vi "Autonomous Independent.vi"() -> ()   [LabVIEW 2017]
doc: "This VI is called when autonomous begins, and will automatically be terminated when autonomous ends. You can carry out timed or sensor driven robot movement independently without needing to return to the caller."
uses:
  Auto Movement Cluster.ctl
  Begin Cluster.ctl
  <vilib>/Rock Robotics/WPI/Encoder/WPI_EncoderDevRef.ctl
  <vilib>/Rock Robotics/SystemInterfaces/Encoder/FPGA_EncoderIdx.ctl
  <vilib>/Rock Robotics/SystemInterfaces/Counter/FPGA_CounterCtrSystemIndex.ctl
  <vilib>/Rock Robotics/WPI/Encoder/WPI_EncoderType.ctl
  <vilib>/Rock Robotics/WPI/Solenoid/WPI_SolenoidDevRef.ctl
  <vilib>/Rock Robotics/WPI/Solenoid/WPI_SolenoidChannel.ctl
  <vilib>/Rock Robotics/WPI/Potentiometer/WPI_PotentiometerDevRef.ctl
  <vilib>/Rock Robotics/SystemInterfaces/AI/FPGA_AIChannel.ctl
  <vilib>/Rock Robotics/WPI/Gyro/WPI_GyroDevRef.ctl
  <vilib>/Rock Robotics/SystemInterfaces/spilib/spi_bus.ctl
  <vilib>/Rock Robotics/WPI/RobotDrive/WPI_RobotDriveDevRef.ctl
  <vilib>/Rock Robotics/WPI/MotorControl/WPI_MotorControlDeviceRef.ctl
  <vilib>/Rock Robotics/WPI/MotorControl/WPI_MotorControlType.ctl
  <vilib>/Rock Robotics/SystemInterfaces/DIO/FPGA_DIOPWMChannel.ctl
  <vilib>/Rock Robotics/WPI/PWM/WPI_PWMDeadband.ctl
  <vilib>/Rock Robotics/SystemInterfaces/DIO/FPGA_DIOChannel.ctl
  <vilib>/Rock Robotics/WPI/Joystick/WPI_JoystickDevRef.ctl
  <vilib>/Rock Robotics/WPI/Joystick/WPI_JoystickDeviceEnum.ctl
  <vilib>/Rock Robotics/WPI/Utilities/WPI_GetSetVariantRefNum.vi
  <vilib>/Rock Robotics/Network Tables/NT Read Number.vi
  Global Variables.vi
  <vilib>/Rock Robotics/Network Tables/NT Read Boolean.vi
  <vilib>/Rock Robotics/WPI/RobotDrive/WPI_RobotDriveArcadeDrive_Standard(NoSaturation).vi
panel:
  in  "SO - Switch & Scale":T1[](array[typedef])=[{"Drive "=-190.0, "Turn"=0.0, "Wait in ms"=0.0, "Turn?"=FALSE, "Wait?"=FALSE, "Align?"=FALSE, "Wait/Turn Drive Power"=0.0, "Wait Turn Power"=0.0, "Elevator Setpoint"=40.0, "Linear Actuator Length"=0.62, "Intake State 2"=enum."Off"}, {"Drive "=0.0, "Turn"=-90.0, "Wait in ms"=0.0, "Turn?"=TRUE, "Wait?"=FALSE, "Align?"=FALSE, "Wait/Turn Drive Power"=0.0, "Wait Turn Power"=0.0, "Elevator Setpoint"=40.0, "Linear Actuator Length"=0.33, "Intake State 2"=enum."Off"}, {"Drive "=60.0, "Turn"=-90.0, "Wait in ms"=0.0, "Turn?"=FALSE, "Wait?"=FALSE, "Align?"=FALSE, "Wait/Turn Drive Power"=0.0, "Wait Turn Power"=0.0, "Elevator Setpoint"=40.0, "Linear Actuator Length"=0.33, "Intake State 2"=enum."Off"}, {"Drive "=0.0, "Turn"=0.0, "Wait in ms"=0.0, "Turn?"=TRUE, "Wait?"=FALSE, "Align?"=FALSE, "Wait/Turn Drive Power"=0.0, "Wait Turn Power"=0.0, "Elevator Setpoint"=40.0, "Linear Actuator Length"=0.33, "Intake State 2"=enum."Off"}, {"Drive "=0.0, "Turn"=0.0, "Wait in ms"=750.0, "Turn?"=FALSE, "Wait?"=TRUE, "Align?"=FALSE, "Wait/Turn Drive Power"=-0.5, "Wait Turn Power"=0.0, "Elevator Setpoint"=40.0, "Linear Actuator Length"=0.33, "Intake State 2"=enum."Off"}, {"Drive "=0.0, "Turn"=0.0, "Wait in ms"=500.0, "Turn?"=FALSE, "Wait?"=TRUE, "Align?"=FALSE, "Wait/Turn Drive Power"=0.0, "Wait Turn Power"=0.0, "Elevator Setpoint"=40.0, "Linear Actuator Length"=0.33, "Intake State 2"=enum."Spit High"}, {"Drive "=-50.0, "Turn"=-0.0, "Wait in ms"=0.0, "Turn?"=FALSE, "Wait?"=FALSE, "Align?"=FALSE, "Wait/Turn Drive Power"=0.0, "Wait Turn Power"=0.0, "Elevator Setpoint"=30.0, "Linear Actuator Length"=0.62, "Intake State 2"=enum."Off"}, {"Drive "=0.0, "Turn"=0.0, "Wait in ms"=1500.0, "Turn?"=FALSE, "Wait?"=FALSE, "Align?"=TRUE, "Wait/Turn Drive Power"=-0.5, "Wait Turn Power"=0.0, "Elevator Setpoint"=1.0, "Linear Actuator Length"=0.62, "Intake State 2"=enum."Intake"}, {"Drive "=-40.0, "Turn"=-0.0, "Wait in ms"=0.0, "Turn?"=FALSE, "Wait?"=FALSE, "Align?"=FALSE, "Wait/Turn Drive Power"=0.0, "Wait Turn Power"=0.0, "Elevator Setpoint"=40.0, "Linear Actuator Length"=0.92, "Intake State 2"=enum."Off"}, {"Drive "=0.0, "Turn"=-90.0, "Wait in ms"=0.0, "Turn?"=TRUE, "Wait?"=FALSE, "Align?"=FALSE, "Wait/Turn Drive Power"=0.0, "Wait Turn Power"=0.0, "Elevator Setpoint"=40.0, "Linear Actuator Length"=0.92, "Intake State 2"=enum."Off"}, {"Drive "=190.0, "Turn"=-90.0, "Wait in ms"=0.0, "Turn?"=FALSE, "Wait?"=FALSE, "Align?"=FALSE, "Wait/Turn Drive Power"=0.0, "Wait Turn Power"=0.0, "Elevator Setpoint"=40.0, "Linear Actuator Length"=0.92, "Intake State 2"=enum."Off"}, {"Drive "=0.0, "Turn"=-30.0, "Wait in ms"=0.0, "Turn?"=TRUE, "Wait?"=FALSE, "Align?"=FALSE, "Wait/Turn Drive Power"=0.2, "Wait Turn Power"=0.0, "Elevator Setpoint"=71.0, "Linear Actuator Length"=0.62, "Intake State 2"=enum."Off"}, {"Drive "=-30.0, "Turn"=-30.0, "Wait in ms"=0.0, "Turn?"=FALSE, "Wait?"=FALSE, "Align?"=FALSE, "Wait/Turn Drive Power"=0.0, "Wait Turn Power"=0.0, "Elevator Setpoint"=71.5, "Linear Actuator Length"=0.62, "Intake State 2"=enum."Off"}, {"Drive "=0.0, "Turn"=0.0, "Wait in ms"=500.0, "Turn?"=FALSE, "Wait?"=TRUE, "Align?"=FALSE, "Wait/Turn Drive Power"=0.0, "Wait Turn Power"=0.0, "Elevator Setpoint"=71.5, "Linear Actuator Length"=0.62, "Intake State 2"=enum."Spit High"}]
  in  "OS - Switch & Scale":T1[](array[typedef])=[{"Drive "=-235.0, "Turn"=0.0, "Wait in ms"=0.0, "Turn?"=FALSE, "Wait?"=FALSE, "Align?"=FALSE, "Wait/Turn Drive Power"=0.0, "Wait Turn Power"=0.0, "Elevator Setpoint"=40.0, "Linear Actuator Length"=0.62, "Intake State 2"=enum."Off"}, {"Drive "=0.0, "Turn"=20.0, "Wait in ms"=0.0, "Turn?"=TRUE, "Wait?"=FALSE, "Align?"=FALSE, "Wait/Turn Drive Power"=0.0, "Wait Turn Power"=0.0, "Elevator Setpoint"=70.0, "Linear Actuator Length"=0.62, "Intake State 2"=enum."Off"}, {"Drive "=-30.0, "Turn"=30.0, "Wait in ms"=0.0, "Turn?"=FALSE, "Wait?"=FALSE, "Align?"=FALSE, "Wait/Turn Drive Power"=0.0, "Wait Turn Power"=0.0, "Elevator Setpoint"=71.5, "Linear Actuator Length"=0.62, "Intake State 2"=enum."Off"}, {"Drive "=0.0, "Turn"=0.0, "Wait in ms"=250.0, "Turn?"=FALSE, "Wait?"=TRUE, "Align?"=FALSE, "Wait/Turn Drive Power"=0.0, "Wait Turn Power"=0.0, "Elevator Setpoint"=71.5, "Linear Actuator Length"=0.62, "Intake State 2"=enum."Spit High"}, {"Drive "=0.0, "Turn"=-20.0, "Wait in ms"=0.0, "Turn?"=TRUE, "Wait?"=FALSE, "Align?"=FALSE, "Wait/Turn Drive Power"=0.0, "Wait Turn Power"=0.0, "Elevator Setpoint"=71.5, "Linear Actuator Length"=0.62, "Intake State 2"=enum."Off"}, {"Drive "=40.0, "Turn"=-20.0, "Wait in ms"=0.0, "Turn?"=FALSE, "Wait?"=FALSE, "Align?"=FALSE, "Wait/Turn Drive Power"=0.0, "Wait Turn Power"=0.0, "Elevator Setpoint"=1.0, "Linear Actuator Length"=0.62, "Intake State 2"=enum."Off"}, {"Drive "=0.0, "Turn"=0.0, "Wait in ms"=1500.0, "Turn?"=FALSE, "Wait?"=FALSE, "Align?"=TRUE, "Wait/Turn Drive Power"=-0.5, "Wait Turn Power"=0.0, "Elevator Setpoint"=1.0, "Linear Actuator Length"=0.62, "Intake State 2"=enum."Intake"}, {"Drive "=-50.0, "Turn"=0.0, "Wait in ms"=0.0, "Turn?"=FALSE, "Wait?"=FALSE, "Align?"=FALSE, "Wait/Turn Drive Power"=0.0, "Wait Turn Power"=0.0, "Elevator Setpoint"=40.0, "Linear Actuator Length"=0.62, "Intake State 2"=enum."Off"}, {"Drive "=0.0, "Turn"=-90.0, "Wait in ms"=0.0, "Turn?"=TRUE, "Wait?"=FALSE, "Align?"=FALSE, "Wait/Turn Drive Power"=0.0, "Wait Turn Power"=0.0, "Elevator Setpoint"=40.0, "Linear Actuator Length"=0.62, "Intake State 2"=enum."Off"}, {"Drive "=165.0, "Turn"=-90.0, "Wait in ms"=0.0, "Turn?"=FALSE, "Wait?"=FALSE, "Align?"=FALSE, "Wait/Turn Drive Power"=0.0, "Wait Turn Power"=0.0, "Elevator Setpoint"=40.0, "Linear Actuator Length"=0.62, "Intake State 2"=enum."Off"}, {"Drive "=0.0, "Turn"=0.0, "Wait in ms"=0.0, "Turn?"=TRUE, "Wait?"=FALSE, "Align?"=FALSE, "Wait/Turn Drive Power"=0.0, "Wait Turn Power"=0.0, "Elevator Setpoint"=40.0, "Linear Actuator Length"=0.33, "Intake State 2"=enum."Off"}, {"Drive "=0.0, "Turn"=0.0, "Wait in ms"=1250.0, "Turn?"=FALSE, "Wait?"=TRUE, "Align?"=FALSE, "Wait/Turn Drive Power"=-0.5, "Wait Turn Power"=0.0, "Elevator Setpoint"=40.0, "Linear Actuator Length"=0.33, "Intake State 2"=enum."Off"}, {"Drive "=0.0, "Turn"=0.0, "Wait in ms"=500.0, "Turn?"=FALSE, "Wait?"=TRUE, "Align?"=FALSE, "Wait/Turn Drive Power"=0.0, "Wait Turn Power"=0.0, "Elevator Setpoint"=40.0, "Linear Actuator Length"=0.33, "Intake State 2"=enum."Spit High"}]
  in  "SS - Switch & Scale":T1[](array[typedef])=[{"Drive "=-235.0, "Turn"=0.0, "Wait in ms"=0.0, "Turn?"=FALSE, "Wait?"=FALSE, "Align?"=FALSE, "Wait/Turn Drive Power"=0.0, "Wait Turn Power"=0.0, "Elevator Setpoint"=40.0, "Linear Actuator Length"=0.62, "Intake State 2"=enum."Off"}, {"Drive "=0.0, "Turn"=20.0, "Wait in ms"=0.0, "Turn?"=TRUE, "Wait?"=FALSE, "Align?"=FALSE, "Wait/Turn Drive Power"=0.0, "Wait Turn Power"=0.0, "Elevator Setpoint"=70.0, "Linear Actuator Length"=0.62, "Intake State 2"=enum."Off"}, {"Drive "=-30.0, "Turn"=30.0, "Wait in ms"=0.0, "Turn?"=FALSE, "Wait?"=FALSE, "Align?"=FALSE, "Wait/Turn Drive Power"=0.0, "Wait Turn Power"=0.0, "Elevator Setpoint"=71.5, "Linear Actuator Length"=0.62, "Intake State 2"=enum."Off"}, {"Drive "=0.0, "Turn"=0.0, "Wait in ms"=250.0, "Turn?"=FALSE, "Wait?"=TRUE, "Align?"=FALSE, "Wait/Turn Drive Power"=0.0, "Wait Turn Power"=0.0, "Elevator Setpoint"=71.5, "Linear Actuator Length"=0.62, "Intake State 2"=enum."Spit High"}, {"Drive "=0.0, "Turn"=-20.0, "Wait in ms"=0.0, "Turn?"=TRUE, "Wait?"=FALSE, "Align?"=FALSE, "Wait/Turn Drive Power"=0.0, "Wait Turn Power"=0.0, "Elevator Setpoint"=71.5, "Linear Actuator Length"=0.62, "Intake State 2"=enum."Off"}, {"Drive "=40.0, "Turn"=-20.0, "Wait in ms"=0.0, "Turn?"=FALSE, "Wait?"=FALSE, "Align?"=FALSE, "Wait/Turn Drive Power"=0.0, "Wait Turn Power"=0.0, "Elevator Setpoint"=1.0, "Linear Actuator Length"=0.62, "Intake State 2"=enum."Off"}, {"Drive "=0.0, "Turn"=0.0, "Wait in ms"=1500.0, "Turn?"=FALSE, "Wait?"=FALSE, "Align?"=TRUE, "Wait/Turn Drive Power"=-0.5, "Wait Turn Power"=0.0, "Elevator Setpoint"=1.0, "Linear Actuator Length"=0.62, "Intake State 2"=enum."Intake"}, {"Drive "=-20.0, "Turn"=0.0, "Wait in ms"=0.0, "Turn?"=FALSE, "Wait?"=FALSE, "Align?"=FALSE, "Wait/Turn Drive Power"=0.0, "Wait Turn Power"=0.0, "Elevator Setpoint"=40.0, "Linear Actuator Length"=0.62, "Intake State 2"=enum."Off"}, {"Drive "=0.0, "Turn"=0.0, "Wait in ms"=750.0, "Turn?"=FALSE, "Wait?"=TRUE, "Align?"=FALSE, "Wait/Turn Drive Power"=-0.5, "Wait Turn Power"=0.0, "Elevator Setpoint"=40.0, "Linear Actuator Length"=0.62, "Intake State 2"=enum."Off"}, {"Drive "=0.0, "Turn"=0.0, "Wait in ms"=500.0, "Turn?"=FALSE, "Wait?"=TRUE, "Align?"=FALSE, "Wait/Turn Drive Power"=0.0, "Wait Turn Power"=0.0, "Elevator Setpoint"=40.0, "Linear Actuator Length"=0.62, "Intake State 2"=enum."Spit High"}]
  in  "OO - Switch & Scale":T1[](array[typedef])=[{"Drive "=-195.0, "Turn"=0.0, "Wait in ms"=0.0, "Turn?"=FALSE, "Wait?"=FALSE, "Align?"=FALSE, "Wait/Turn Drive Power"=0.0, "Wait Turn Power"=0.0, "Elevator Setpoint"=40.0, "Linear Actuator Length"=0.92, "Intake State 2"=enum."Off"}, {"Drive "=0.0, "Turn"=-90.0, "Wait in ms"=0.0, "Turn?"=TRUE, "Wait?"=FALSE, "Align?"=FALSE, "Wait/Turn Drive Power"=0.0, "Wait Turn Power"=0.0, "Elevator Setpoint"=40.0, "Linear Actuator Length"=0.92, "Intake State 2"=enum."Off"}, {"Drive "=200.0, "Turn"=-90.0, "Wait in ms"=0.0, "Turn?"=FALSE, "Wait?"=FALSE, "Align?"=FALSE, "Wait/Turn Drive Power"=0.0, "Wait Turn Power"=0.0, "Elevator Setpoint"=40.0, "Linear Actuator Length"=0.92, "Intake State 2"=enum."Off"}, {"Drive "=0.0, "Turn"=-30.0, "Wait in ms"=0.0, "Turn?"=TRUE, "Wait?"=FALSE, "Align?"=FALSE, "Wait/Turn Drive Power"=0.2, "Wait Turn Power"=0.0, "Elevator Setpoint"=71.0, "Linear Actuator Length"=0.92, "Intake State 2"=enum."Off"}, {"Drive "=-30.0, "Turn"=-30.0, "Wait in ms"=0.0, "Turn?"=FALSE, "Wait?"=FALSE, "Align?"=FALSE, "Wait/Turn Drive Power"=0.0, "Wait Turn Power"=0.0, "Elevator Setpoint"=71.5, "Linear Actuator Length"=0.62, "Intake State 2"=enum."Off"}, {"Drive "=0.0, "Turn"=0.0, "Wait in ms"=500.0, "Turn?"=FALSE, "Wait?"=TRUE, "Align?"=FALSE, "Wait/Turn Drive Power"=0.0, "Wait Turn Power"=0.0, "Elevator Setpoint"=71.5, "Linear Actuator Length"=0.62, "Intake State 2"=enum."Spit Low"}, {"Drive "=0.0, "Turn"=10.0, "Wait in ms"=0.0, "Turn?"=TRUE, "Wait?"=FALSE, "Align?"=FALSE, "Wait/Turn Drive Power"=0.0, "Wait Turn Power"=0.0, "Elevator Setpoint"=71.5, "Linear Actuator Length"=0.62, "Intake State 2"=enum."Off"}, {"Drive "=30.0, "Turn"=10.0, "Wait in ms"=0.0, "Turn?"=FALSE, "Wait?"=FALSE, "Align?"=FALSE, "Wait/Turn Drive Power"=0.0, "Wait Turn Power"=0.0, "Elevator Setpoint"=1.0, "Linear Actuator Length"=0.62, "Intake State 2"=enum."Off"}, {"Drive "=0.0, "Turn"=0.0, "Wait in ms"=1500.0, "Turn?"=FALSE, "Wait?"=FALSE, "Align?"=TRUE, "Wait/Turn Drive Power"=0.0, "Wait Turn Power"=0.0, "Elevator Setpoint"=1.0, "Linear Actuator Length"=0.62, "Intake State 2"=enum."Intake"}, {"Drive "=-20.0, "Turn"=0.0, "Wait in ms"=0.0, "Turn?"=FALSE, "Wait?"=FALSE, "Align?"=FALSE, "Wait/Turn Drive Power"=0.0, "Wait Turn Power"=0.0, "Elevator Setpoint"=40.0, "Linear Actuator Length"=0.62, "Intake State 2"=enum."Off"}, {"Drive "=0.0, "Turn"=0.0, "Wait in ms"=750.0, "Turn?"=FALSE, "Wait?"=TRUE, "Align?"=FALSE, "Wait/Turn Drive Power"=-0.5, "Wait Turn Power"=0.0, "Elevator Setpoint"=40.0, "Linear Actuator Length"=0.62, "Intake State 2"=enum."Off"}, {"Drive "=0.0, "Turn"=0.0, "Wait in ms"=500.0, "Turn?"=FALSE, "Wait?"=TRUE, "Align?"=FALSE, "Wait/Turn Drive Power"=0.0, "Wait Turn Power"=0.0, "Elevator Setpoint"=40.0, "Linear Actuator Length"=0.62, "Intake State 2"=enum."Spit High"}]
  in  "Middle Switch One":T1[](array[typedef])=[{"Drive "=20.0, "Turn"=0.0, "Wait in ms"=0.0, "Turn?"=FALSE, "Wait?"=FALSE, "Align?"=FALSE, "Wait/Turn Drive Power"=0.0, "Wait Turn Power"=0.0, "Elevator Setpoint"=30.0, "Linear Actuator Length"=0.62, "Intake State 2"=enum."Off"}, {"Drive "=0.0, "Turn"=-40.0, "Wait in ms"=0.0, "Turn?"=TRUE, "Wait?"=FALSE, "Align?"=FALSE, "Wait/Turn Drive Power"=-0.1, "Wait Turn Power"=0.0, "Elevator Setpoint"=30.0, "Linear Actuator Length"=0.62, "Intake State 2"=enum."Off"}, {"Drive "=80.0, "Turn"=-40.0, "Wait in ms"=0.0, "Turn?"=FALSE, "Wait?"=FALSE, "Align?"=FALSE, "Wait/Turn Drive Power"=0.0, "Wait Turn Power"=0.0, "Elevator Setpoint"=30.0, "Linear Actuator Length"=0.62, "Intake State 2"=enum."Off"}, {"Drive "=0.0, "Turn"=0.0, "Wait in ms"=0.0, "Turn?"=TRUE, "Wait?"=FALSE, "Align?"=FALSE, "Wait/Turn Drive Power"=-0.5, "Wait Turn Power"=0.0, "Elevator Setpoint"=30.0, "Linear Actuator Length"=0.62, "Intake State 2"=enum."Off"}, {"Drive "=0.0, "Turn"=0.0, "Wait in ms"=900.0, "Turn?"=FALSE, "Wait?"=TRUE, "Align?"=FALSE, "Wait/Turn Drive Power"=-0.5, "Wait Turn Power"=0.0, "Elevator Setpoint"=30.0, "Linear Actuator Length"=0.62, "Intake State 2"=enum."Off"}, {"Drive "=0.0, "Turn"=0.0, "Wait in ms"=250.0, "Turn?"=FALSE, "Wait?"=TRUE, "Align?"=FALSE, "Wait/Turn Drive Power"=-0.2, "Wait Turn Power"=0.0, "Elevator Setpoint"=30.0, "Linear Actuator Length"=0.62, "Intake State 2"=enum."Spit High"}]
  in  "Cross":T1[](array[typedef])=[{"Drive "=-210.0, "Turn"=0.0, "Wait in ms"=0.0, "Turn?"=FALSE, "Wait?"=FALSE, "Align?"=FALSE, "Wait/Turn Drive Power"=0.0, "Wait Turn Power"=0.0, "Elevator Setpoint"=40.0, "Linear Actuator Length"=0.92, "Intake State 2"=enum."Off"}, {"Drive "=0.0, "Turn"=-90.0, "Wait in ms"=0.0, "Turn?"=TRUE, "Wait?"=FALSE, "Align?"=FALSE, "Wait/Turn Drive Power"=0.0, "Wait Turn Power"=0.0, "Elevator Setpoint"=40.0, "Linear Actuator Length"=0.92, "Intake State 2"=enum."Off"}, {"Drive "=36.0, "Turn"=-90.0, "Wait in ms"=0.0, "Turn?"=FALSE, "Wait?"=FALSE, "Align?"=FALSE, "Wait/Turn Drive Power"=0.0, "Wait Turn Power"=0.0, "Elevator Setpoint"=40.0, "Linear Actuator Length"=0.92, "Intake State 2"=enum."Off"}, {"Drive "=0.0, "Turn"=0.0, "Wait in ms"=0.0, "Turn?"=FALSE, "Wait?"=FALSE, "Align?"=FALSE, "Wait/Turn Drive Power"=0.0, "Wait Turn Power"=0.0, "Elevator Setpoint"=40.0, "Linear Actuator Length"=0.92, "Intake State 2"=enum."Off"}]
  in  "Do Nothing":T1[](array[typedef])=[{"Drive "=0.0, "Turn"=0.0, "Wait in ms"=0.0, "Turn?"=FALSE, "Wait?"=FALSE, "Align?"=FALSE, "Wait/Turn Drive Power"=0.0, "Wait Turn Power"=0.0, "Elevator Setpoint"=35.0, "Linear Actuator Length"=0.65, "Intake State 2"=enum."Off"}]
  in  "Outer Scale":T1[](array[typedef])=[{"Drive "=-310.0, "Turn"=0.0, "Wait in ms"=0.0, "Turn?"=FALSE, "Wait?"=FALSE, "Align?"=FALSE, "Wait/Turn Drive Power"=0.0, "Wait Turn Power"=0.0, "Elevator Setpoint"=40.0, "Linear Actuator Length"=0.62, "Intake State 2"=enum."Off"}, {"Drive "=0.0, "Turn"=90.0, "Wait in ms"=0.0, "Turn?"=TRUE, "Wait?"=FALSE, "Align?"=FALSE, "Wait/Turn Drive Power"=0.0, "Wait Turn Power"=0.0, "Elevator Setpoint"=70.0, "Linear Actuator Length"=0.62, "Intake State 2"=enum."Off"}, {"Drive "=-30.0, "Turn"=90.0, "Wait in ms"=0.0, "Turn?"=FALSE, "Wait?"=FALSE, "Align?"=FALSE, "Wait/Turn Drive Power"=0.0, "Wait Turn Power"=0.0, "Elevator Setpoint"=71.5, "Linear Actuator Length"=0.62, "Intake State 2"=enum."Off"}, {"Drive "=0.0, "Turn"=90.0, "Wait in ms"=500.0, "Turn?"=FALSE, "Wait?"=TRUE, "Align?"=FALSE, "Wait/Turn Drive Power"=0.0, "Wait Turn Power"=0.0, "Elevator Setpoint"=71.5, "Linear Actuator Length"=0.62, "Intake State 2"=enum."Spit High"}, {"Drive "=40.0, "Turn"=90.0, "Wait in ms"=0.0, "Turn?"=FALSE, "Wait?"=FALSE, "Align?"=FALSE, "Wait/Turn Drive Power"=0.0, "Wait Turn Power"=0.0, "Elevator Setpoint"=71.5, "Linear Actuator Length"=0.62, "Intake State 2"=enum."Off"}, {"Drive "=0.0, "Turn"=200.0, "Wait in ms"=0.0, "Turn?"=TRUE, "Wait?"=FALSE, "Align?"=FALSE, "Wait/Turn Drive Power"=0.0, "Wait Turn Power"=0.0, "Elevator Setpoint"=40.0, "Linear Actuator Length"=0.92, "Intake State 2"=enum."Off"}]
  in  "Middle Switch Two":T1[](array[typedef])=[{"Drive "=20.0, "Turn"=0.0, "Wait in ms"=0.0, "Turn?"=FALSE, "Wait?"=FALSE, "Align?"=FALSE, "Wait/Turn Drive Power"=0.0, "Wait Turn Power"=0.0, "Elevator Setpoint"=30.0, "Linear Actuator Length"=0.62, "Intake State 2"=enum."Off"}, {"Drive "=0.0, "Turn"=-40.0, "Wait in ms"=0.0, "Turn?"=TRUE, "Wait?"=FALSE, "Align?"=FALSE, "Wait/Turn Drive Power"=-0.1, "Wait Turn Power"=0.0, "Elevator Setpoint"=30.0, "Linear Actuator Length"=0.62, "Intake State 2"=enum."Off"}, {"Drive "=80.0, "Turn"=-40.0, "Wait in ms"=0.0, "Turn?"=FALSE, "Wait?"=FALSE, "Align?"=FALSE, "Wait/Turn Drive Power"=0.0, "Wait Turn Power"=0.0, "Elevator Setpoint"=30.0, "Linear Actuator Length"=0.62, "Intake State 2"=enum."Off"}, {"Drive "=0.0, "Turn"=0.0, "Wait in ms"=0.0, "Turn?"=TRUE, "Wait?"=FALSE, "Align?"=FALSE, "Wait/Turn Drive Power"=-0.5, "Wait Turn Power"=0.0, "Elevator Setpoint"=30.0, "Linear Actuator Length"=0.62, "Intake State 2"=enum."Off"}, {"Drive "=0.0, "Turn"=0.0, "Wait in ms"=900.0, "Turn?"=FALSE, "Wait?"=TRUE, "Align?"=FALSE, "Wait/Turn Drive Power"=-0.5, "Wait Turn Power"=0.0, "Elevator Setpoint"=30.0, "Linear Actuator Length"=0.62, "Intake State 2"=enum."Off"}, {"Drive "=0.0, "Turn"=0.0, "Wait in ms"=250.0, "Turn?"=FALSE, "Wait?"=TRUE, "Align?"=FALSE, "Wait/Turn Drive Power"=-0.2, "Wait Turn Power"=0.0, "Elevator Setpoint"=30.0, "Linear Actuator Length"=0.62, "Intake State 2"=enum."Spit High"}, {"Drive "=-60.0, "Turn"=0.0, "Wait in ms"=0.0, "Turn?"=FALSE, "Wait?"=FALSE, "Align?"=FALSE, "Wait/Turn Drive Power"=0.0, "Wait Turn Power"=0.0, "Elevator Setpoint"=30.0, "Linear Actuator Length"=0.62, "Intake State 2"=enum."Off"}, {"Drive "=0.0, "Turn"=25.0, "Wait in ms"=0.0, "Turn?"=TRUE, "Wait?"=FALSE, "Align?"=FALSE, "Wait/Turn Drive Power"=0.0, "Wait Turn Power"=0.0, "Elevator Setpoint"=1.0, "Linear Actuator Length"=0.62, "Intake State 2"=enum."Off"}, {"Drive "=0.0, "Turn"=0.0, "Wait in ms"=2500.0, "Turn?"=FALSE, "Wait?"=TRUE, "Align?"=FALSE, "Wait/Turn Drive Power"=-0.5, "Wait Turn Power"=0.0, "Elevator Setpoint"=1.0, "Linear Actuator Length"=0.62, "Intake State 2"=enum."Intake"}, {"Drive "=0.0, "Turn"=0.0, "Wait in ms"=250.0, "Turn?"=FALSE, "Wait?"=TRUE, "Align?"=FALSE, "Wait/Turn Drive Power"=0.3, "Wait Turn Power"=0.0, "Elevator Setpoint"=1.0, "Linear Actuator Length"=0.62, "Intake State 2"=enum."Intake"}, {"Drive "=-40.0, "Turn"=45.0, "Wait in ms"=0.0, "Turn?"=FALSE, "Wait?"=FALSE, "Align?"=FALSE, "Wait/Turn Drive Power"=0.0, "Wait Turn Power"=0.0, "Elevator Setpoint"=30.0, "Linear Actuator Length"=0.62, "Intake State 2"=enum."Off"}, {"Drive "=0.0, "Turn"=0.0, "Wait in ms"=0.0, "Turn?"=TRUE, "Wait?"=FALSE, "Align?"=FALSE, "Wait/Turn Drive Power"=0.0, "Wait Turn Power"=0.0, "Elevator Setpoint"=30.0, "Linear Actuator Length"=0.62, "Intake State 2"=enum."Off"}, {"Drive "=0.0, "Turn"=0.0, "Wait in ms"=1500.0, "Turn?"=FALSE, "Wait?"=TRUE, "Align?"=FALSE, "Wait/Turn Drive Power"=-0.6, "Wait Turn Power"=0.0, "Elevator Setpoint"=30.0, "Linear Actuator Length"=0.62, "Intake State 2"=enum."Off"}, {"Drive "=0.0, "Turn"=0.0, "Wait in ms"=500.0, "Turn?"=FALSE, "Wait?"=TRUE, "Align?"=FALSE, "Wait/Turn Drive Power"=-0.4, "Wait Turn Power"=0.0, "Elevator Setpoint"=30.0, "Linear Actuator Length"=0.62, "Intake State 2"=enum."Spit High"}]
  in  "O - Scale Only":T1[](array[typedef])=[{"Drive "=-195.0, "Turn"=0.0, "Wait in ms"=0.0, "Turn?"=FALSE, "Wait?"=FALSE, "Align?"=FALSE, "Wait/Turn Drive Power"=0.0, "Wait Turn Power"=0.0, "Elevator Setpoint"=40.0, "Linear Actuator Length"=0.92, "Intake State 2"=enum."Off"}, {"Drive "=0.0, "Turn"=-90.0, "Wait in ms"=0.0, "Turn?"=TRUE, "Wait?"=FALSE, "Align?"=FALSE, "Wait/Turn Drive Power"=0.0, "Wait Turn Power"=0.0, "Elevator Setpoint"=40.0, "Linear Actuator Length"=0.92, "Intake State 2"=enum."Off"}, {"Drive "=200.0, "Turn"=-90.0, "Wait in ms"=0.0, "Turn?"=FALSE, "Wait?"=FALSE, "Align?"=FALSE, "Wait/Turn Drive Power"=0.0, "Wait Turn Power"=0.0, "Elevator Setpoint"=40.0, "Linear Actuator Length"=0.92, "Intake State 2"=enum."Off"}, {"Drive "=0.0, "Turn"=-30.0, "Wait in ms"=0.0, "Turn?"=TRUE, "Wait?"=FALSE, "Align?"=FALSE, "Wait/Turn Drive Power"=0.2, "Wait Turn Power"=0.0, "Elevator Setpoint"=71.0, "Linear Actuator Length"=0.92, "Intake State 2"=enum."Off"}, {"Drive "=-30.0, "Turn"=-30.0, "Wait in ms"=0.0, "Turn?"=FALSE, "Wait?"=FALSE, "Align?"=FALSE, "Wait/Turn Drive Power"=0.0, "Wait Turn Power"=0.0, "Elevator Setpoint"=71.5, "Linear Actuator Length"=0.62, "Intake State 2"=enum."Off"}, {"Drive "=0.0, "Turn"=0.0, "Wait in ms"=500.0, "Turn?"=FALSE, "Wait?"=TRUE, "Align?"=FALSE, "Wait/Turn Drive Power"=0.0, "Wait Turn Power"=0.0, "Elevator Setpoint"=71.5, "Linear Actuator Length"=0.62, "Intake State 2"=enum."Spit High"}, {"Drive "=0.0, "Turn"=10.0, "Wait in ms"=0.0, "Turn?"=TRUE, "Wait?"=FALSE, "Align?"=FALSE, "Wait/Turn Drive Power"=0.0, "Wait Turn Power"=0.0, "Elevator Setpoint"=71.5, "Linear Actuator Length"=0.62, "Intake State 2"=enum."Off"}, {"Drive "=26.0, "Turn"=10.0, "Wait in ms"=0.0, "Turn?"=FALSE, "Wait?"=FALSE, "Align?"=FALSE, "Wait/Turn Drive Power"=0.0, "Wait Turn Power"=0.0, "Elevator Setpoint"=1.0, "Linear Actuator Length"=0.62, "Intake State 2"=enum."Off"}, {"Drive "=0.0, "Turn"=0.0, "Wait in ms"=1500.0, "Turn?"=FALSE, "Wait?"=FALSE, "Align?"=TRUE, "Wait/Turn Drive Power"=0.0, "Wait Turn Power"=0.0, "Elevator Setpoint"=1.0, "Linear Actuator Length"=0.62, "Intake State 2"=enum."Intake"}, {"Drive "=-50.0, "Turn"=10.0, "Wait in ms"=0.0, "Turn?"=FALSE, "Wait?"=FALSE, "Align?"=FALSE, "Wait/Turn Drive Power"=0.0, "Wait Turn Power"=0.0, "Elevator Setpoint"=71.0, "Linear Actuator Length"=0.62, "Intake State 2"=enum."Off"}, {"Drive "=0.0, "Turn"=-30.0, "Wait in ms"=0.0, "Turn?"=TRUE, "Wait?"=FALSE, "Align?"=FALSE, "Wait/Turn Drive Power"=0.0, "Wait Turn Power"=0.0, "Elevator Setpoint"=71.5, "Linear Actuator Length"=0.62, "Intake State 2"=enum."Off"}, {"Drive "=0.0, "Turn"=0.0, "Wait in ms"=500.0, "Turn?"=FALSE, "Wait?"=TRUE, "Align?"=FALSE, "Wait/Turn Drive Power"=0.0, "Wait Turn Power"=0.0, "Elevator Setpoint"=71.5, "Linear Actuator Length"=0.62, "Intake State 2"=enum."Off"}, {"Drive "=0.0, "Turn"=0.0, "Wait in ms"=500.0, "Turn?"=FALSE, "Wait?"=TRUE, "Align?"=FALSE, "Wait/Turn Drive Power"=0.0, "Wait Turn Power"=0.0, "Elevator Setpoint"=71.5, "Linear Actuator Length"=0.62, "Intake State 2"=enum."Spit High"}]
  in  "Quarter Switch Only":T1[](array[typedef])=[{"Drive "=-150.0, "Turn"=0.0, "Wait in ms"=0.0, "Turn?"=FALSE, "Wait?"=FALSE, "Align?"=FALSE, "Wait/Turn Drive Power"=0.0, "Wait Turn Power"=0.0, "Elevator Setpoint"=30.0, "Linear Actuator Length"=0.62, "Intake State 2"=enum."Off"}, {"Drive "=0.0, "Turn"=-90.0, "Wait in ms"=0.0, "Turn?"=TRUE, "Wait?"=FALSE, "Align?"=FALSE, "Wait/Turn Drive Power"=0.0, "Wait Turn Power"=0.0, "Elevator Setpoint"=30.0, "Linear Actuator Length"=0.62, "Intake State 2"=enum."Off"}, {"Drive "=0.0, "Turn"=0.0, "Wait in ms"=250.0, "Turn?"=FALSE, "Wait?"=TRUE, "Align?"=FALSE, "Wait/Turn Drive Power"=-0.7, "Wait Turn Power"=0.0, "Elevator Setpoint"=30.0, "Linear Actuator Length"=0.62, "Intake State 2"=enum."Spit High"}]
  in  "S - Scale Only":T1[](array[typedef])=[{"Drive "=-248.0, "Turn"=0.0, "Wait in ms"=0.0, "Turn?"=FALSE, "Wait?"=FALSE, "Align?"=FALSE, "Wait/Turn Drive Power"=0.0, "Wait Turn Power"=0.0, "Elevator Setpoint"=40.0, "Linear Actuator Length"=0.62, "Intake State 2"=enum."Off"}, {"Drive "=0.0, "Turn"=40.0, "Wait in ms"=0.0, "Turn?"=TRUE, "Wait?"=FALSE, "Align?"=FALSE, "Wait/Turn Drive Power"=0.0, "Wait Turn Power"=0.0, "Elevator Setpoint"=40.0, "Linear Actuator Length"=0.62, "Intake State 2"=enum."Off"}, {"Drive "=0.0, "Turn"=0.0, "Wait in ms"=500.0, "Turn?"=FALSE, "Wait?"=TRUE, "Align?"=FALSE, "Wait/Turn Drive Power"=0.0, "Wait Turn Power"=0.0, "Elevator Setpoint"=70.0, "Linear Actuator Length"=0.62, "Intake State 2"=enum."Off"}, {"Drive "=-22.0, "Turn"=40.0, "Wait in ms"=0.0, "Turn?"=FALSE, "Wait?"=FALSE, "Align?"=FALSE, "Wait/Turn Drive Power"=0.0, "Wait Turn Power"=0.0, "Elevator Setpoint"=71.5, "Linear Actuator Length"=0.62, "Intake State 2"=enum."Off"}, {"Drive "=0.0, "Turn"=0.0, "Wait in ms"=750.0, "Turn?"=FALSE, "Wait?"=TRUE, "Align?"=FALSE, "Wait/Turn Drive Power"=0.0, "Wait Turn Power"=0.0, "Elevator Setpoint"=71.5, "Linear Actuator Length"=0.62, "Intake State 2"=enum."Off"}, {"Drive "=0.0, "Turn"=0.0, "Wait in ms"=500.0, "Turn?"=FALSE, "Wait?"=TRUE, "Align?"=FALSE, "Wait/Turn Drive Power"=0.0, "Wait Turn Power"=0.0, "Elevator Setpoint"=71.5, "Linear Actuator Length"=0.62, "Intake State 2"=enum."Spit High"}, {"Drive "=20.0, "Turn"=40.0, "Wait in ms"=0.0, "Turn?"=FALSE, "Wait?"=FALSE, "Align?"=FALSE, "Wait/Turn Drive Power"=0.0, "Wait Turn Power"=0.0, "Elevator Setpoint"=71.5, "Linear Actuator Length"=0.62, "Intake State 2"=enum."Off"}, {"Drive "=0.0, "Turn"=-28.0, "Wait in ms"=0.0, "Turn?"=TRUE, "Wait?"=FALSE, "Align?"=FALSE, "Wait/Turn Drive Power"=0.0, "Wait Turn Power"=0.0, "Elevator Setpoint"=71.5, "Linear Actuator Length"=0.62, "Intake State 2"=enum."Off"}, {"Drive "=38.0, "Turn"=-28.0, "Wait in ms"=0.0, "Turn?"=FALSE, "Wait?"=FALSE, "Align?"=FALSE, "Wait/Turn Drive Power"=0.0, "Wait Turn Power"=0.0, "Elevator Setpoint"=1.0, "Linear Actuator Length"=0.62, "Intake State 2"=enum."Off"}, {"Drive "=0.0, "Turn"=0.0, "Wait in ms"=750.0, "Turn?"=FALSE, "Wait?"=FALSE, "Align?"=FALSE, "Wait/Turn Drive Power"=0.0, "Wait Turn Power"=0.0, "Elevator Setpoint"=1.0, "Linear Actuator Length"=0.62, "Intake State 2"=enum."Off"}, {"Drive "=0.0, "Turn"=0.0, "Wait in ms"=1000.0, "Turn?"=FALSE, "Wait?"=FALSE, "Align?"=TRUE, "Wait/Turn Drive Power"=-0.5, "Wait Turn Power"=0.0, "Elevator Setpoint"=1.0, "Linear Actuator Length"=0.62, "Intake State 2"=enum."Intake"}, {"Drive "=-60.0, "Turn"=-10.0, "Wait in ms"=0.0, "Turn?"=FALSE, "Wait?"=FALSE, "Align?"=FALSE, "Wait/Turn Drive Power"=0.0, "Wait Turn Power"=0.0, "Elevator Setpoint"=70.0, "Linear Actuator Length"=0.62, "Intake State 2"=enum."Off"}, {"Drive "=0.0, "Turn"=35.0, "Wait in ms"=0.0, "Turn?"=TRUE, "Wait?"=FALSE, "Align?"=FALSE, "Wait/Turn Drive Power"=0.0, "Wait Turn Power"=0.0, "Elevator Setpoint"=71.5, "Linear Actuator Length"=0.62, "Intake State 2"=enum."Off"}, {"Drive "=0.0, "Turn"=0.0, "Wait in ms"=500.0, "Turn?"=FALSE, "Wait?"=TRUE, "Align?"=FALSE, "Wait/Turn Drive Power"=0.0, "Wait Turn Power"=0.0, "Elevator Setpoint"=71.5, "Linear Actuator Length"=0.62, "Intake State 2"=enum."Off"}, {"Drive "=0.0, "Turn"=0.0, "Wait in ms"=500.0, "Turn?"=FALSE, "Wait?"=TRUE, "Align?"=FALSE, "Wait/Turn Drive Power"=0.0, "Wait Turn Power"=0.0, "Elevator Setpoint"=71.5, "Linear Actuator Length"=0.62, "Intake State 2"=enum."Spit High"}]
  # "Be sure to right-click and choose Data Operations>>Make Current Value default if you want to save the array values with the VI"
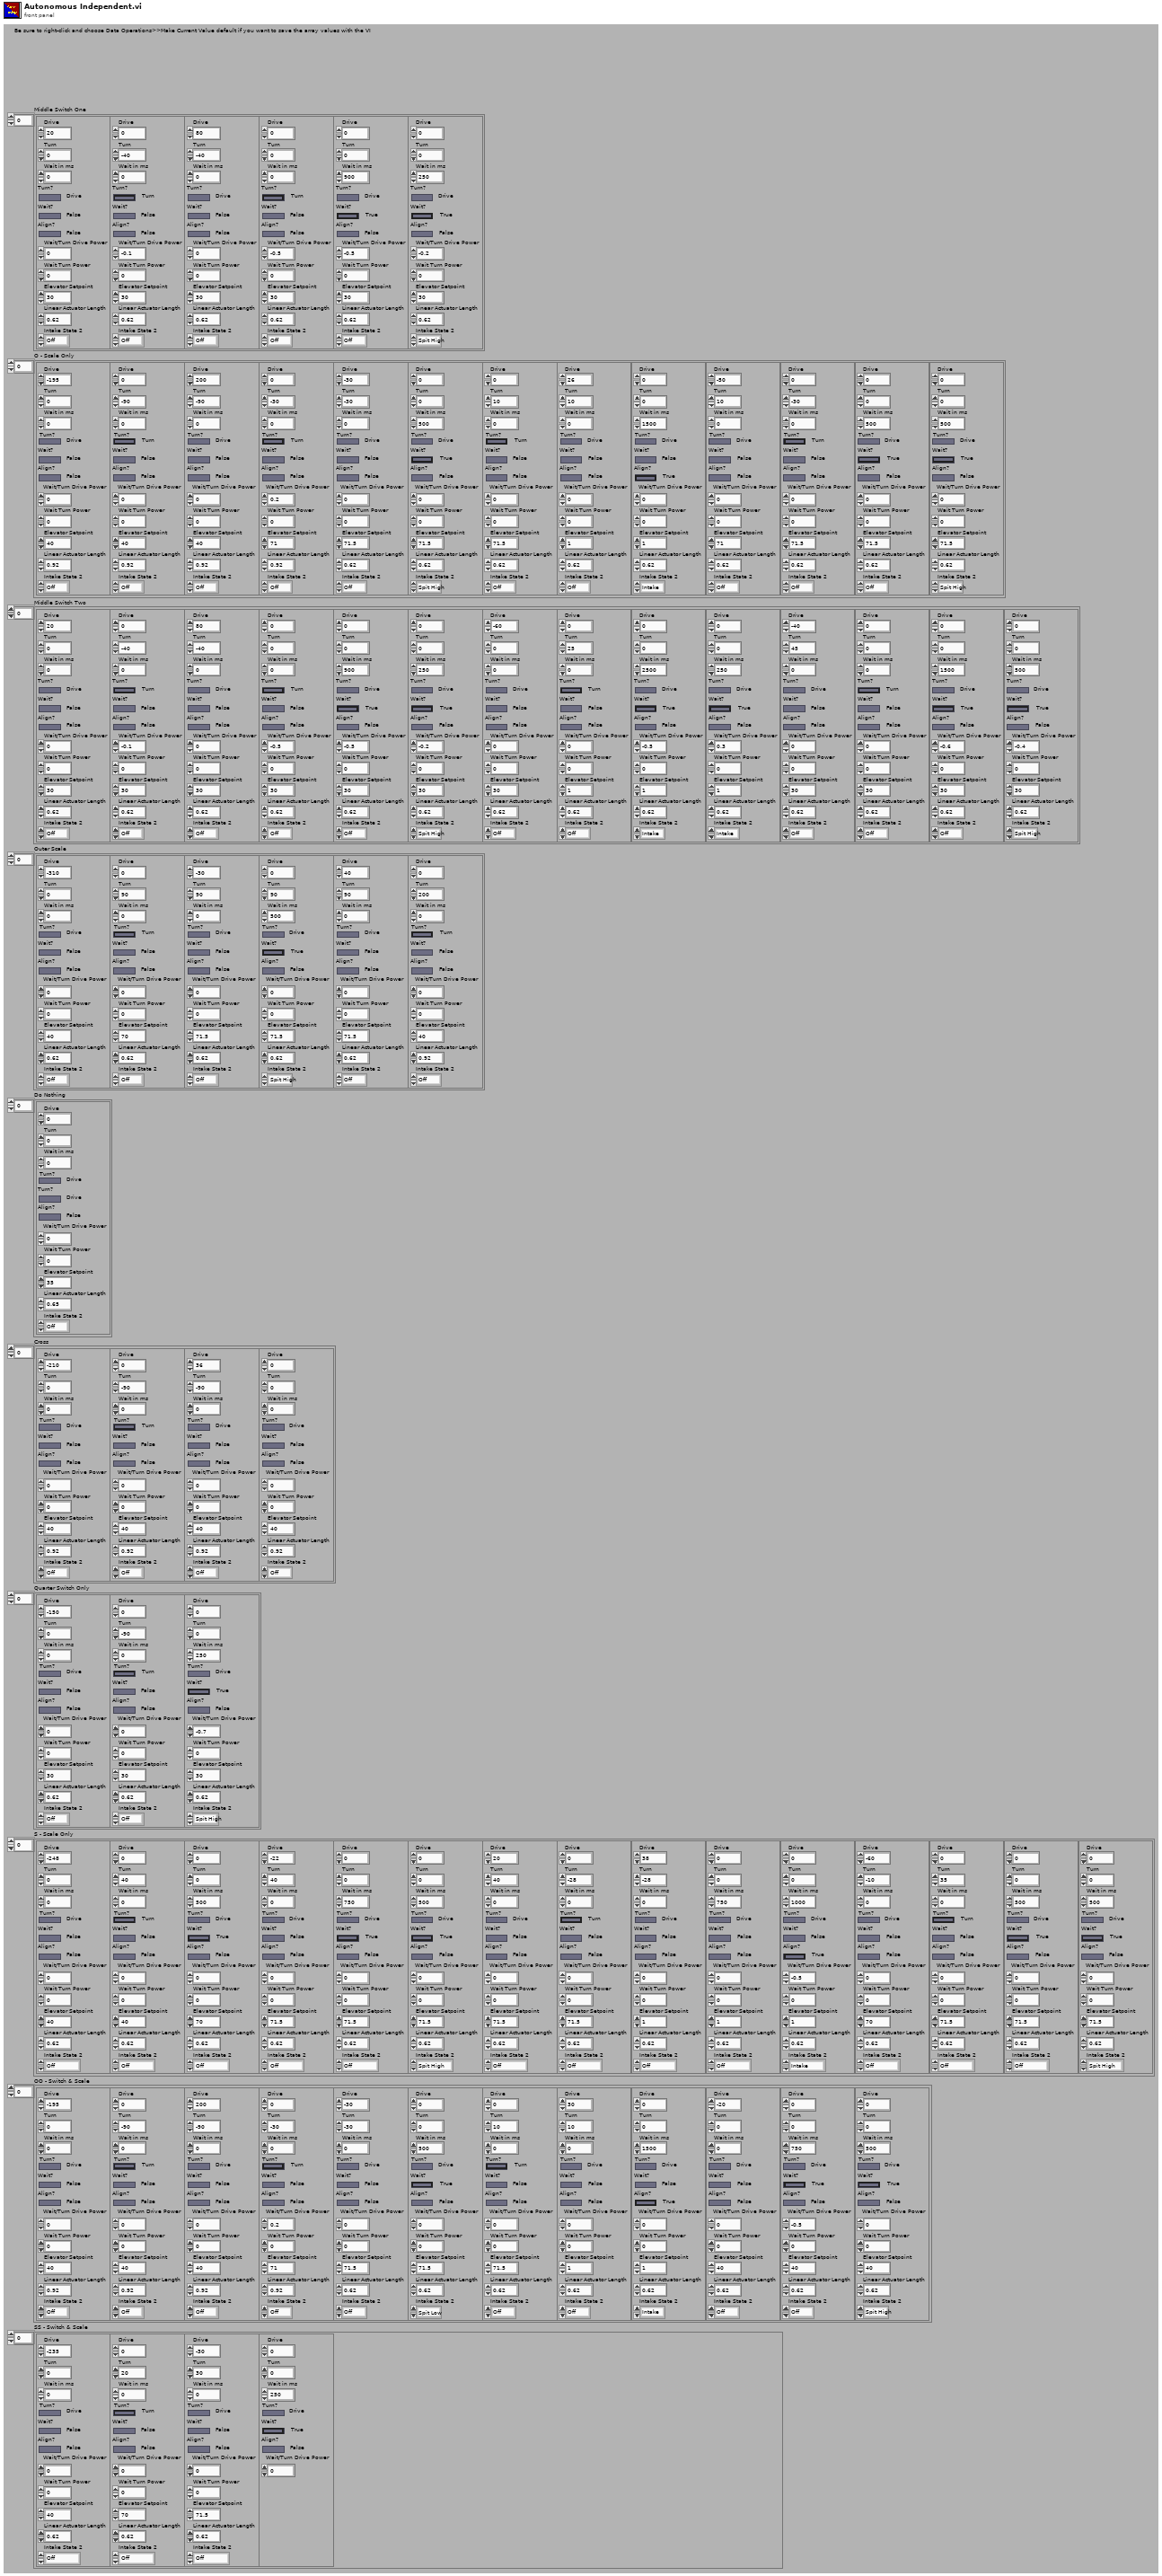
[diagram p1: front panel]
types:
  T1 = typedef "Auto Movement Cluster.ctl" = cluster{"Drive ":dbl, "Turn":dbl, "Wait in ms":dbl, "Turn?":bool, "Wait?":bool, "Align?":bool, "Wait/Turn Drive Power":dbl, "Wait Turn Power":dbl, "Elevator Setpoint":dbl, "Linear Actuator Length":dbl, "Intake State 2":enum16{"Off", "Intake", "Spit Low", "Spit High"}}
  T2 = enum16{"Do Nothing", "Field Open", "Quarter", "Switch Only", "Cross Only"}
  T3 = typedef "Begin Cluster.ctl" = cluster{"Left Drive Encoder":T4, "Right Drive Encoder":T4, "Elevator Encoder":T4, "Drive Shifter":T8, "Elevator Shifter":T8, "Elevator Brake":T8, "Intake Clamp":T8, "Intake Hinge":T8, "Pot Left":T10, "Pot Right":T10, "Gyro":T12, "Drive Motors":T14, "Elevator Master":T15, "Intake Left":T15, "Intake Right":T15, "Linear Actuator Left":T15, "Linear Actuator Right":T15, "X Joystick":T20, "Y Joystick":T20, "Controller":T20, "775 Drive Motors":T14, "Intake Angle Encoder":T4, "Intake Angle":T15}
  T4 = typedef "WPI_EncoderDevRef.ctl" = cluster{"DevStatus":errorcluster, "EncoderIndex":T5, "CounterIndex":T6, "DistancePerCount":dbl, "Decoding Type":T7}
  T5 = typedef "FPGA_EncoderIdx.ctl" = enum8{"Enc 0", "Enc 1", "Enc 2", "Enc 3", "Enc 4", "Enc 5", "Enc 6", "Enc 7", "Invalid"}
  T6 = typedef "FPGA_CounterCtrSystemIndex.ctl" = enum8{"Ctr 0", "Ctr 1", "Ctr 2", "Ctr 3", "Ctr 4", "Ctr 5", "Ctr 6", "Ctr 7", "Invalid"}
  T7 = typedef "WPI_EncoderType.ctl" = enum16{"1x", "2x", "4x"}
  T8 = typedef "WPI_SolenoidDevRef.ctl" = cluster{"DevStatus":errorcluster, "Pneumatics Control Module":u8, "Forward Solenoid Channel":T9, "Reverse Solenoid Channel":T9}
  T9 = typedef "WPI_SolenoidChannel.ctl" = enum8{"Solenoid 0", "Solenoid 1", "Solenoid 2", "Solenoid 3", "Solenoid 4", "Solenoid 5", "Solenoid 6", "Solenoid 7", "Invalid"}
  T10 = typedef "WPI_PotentiometerDevRef.ctl" = cluster{"DevStatus":errorcluster, "Analog Channel":T11, "Invert Output":bool}
  T11 = typedef "FPGA_AIChannel.ctl" = enum8{"AI 0", "AI 1", "AI 2", "AI 3", "AI MXP 0", "AI MXP 1", "AI MXP 2", "AI MXP 3", "Invalid"}
  T12 = typedef "WPI_GyroDevRef.ctl" = cluster{"DevStatus":errorcluster, "Analog Channel":T11, "Gain (VoltsPerDegree/Second)":dbl, "Gyro Type":enum16{"Analog", "XRS450"}, "Handle":i32, "SPI Bus":T13, "Device Found":bool, "Sample Rate":dbl, "Calibrate On Open":bool, "Offset":dbl}
  T13 = typedef "spi_bus.ctl" = enum16{"SPI On-Board, CS0", "SPI On-Board, CS1", "SPI On-Board, CS2", "SPI On-Board, CS3", "SPI MXP", "Invalid"}
  T14 = typedef "WPI_RobotDriveDevRef.ctl" = cluster{"DevStatus":errorcluster, "Motors[]":T15[], "Square Inputs":bool, "Max Output":dbl}
  T15 = typedef "WPI_MotorControlDeviceRef.ctl" = cluster{"DeviceStatus":errorcluster, "Type":T16, "PWM":cluster{"PWM Channel":T17, "DeadBand":T18}, "CAN":cluster{"Device Number":u8, "SetOutput VI Ref":variant, "GetOutput VI Ref":variant, "Enable VI Ref":variant, "Disable VI Ref":variant, "Data":variant}, "Invert":bool, "DIO PWM":cluster{"PWM \"Enable\" Channel":T17, "DIOChannel":T19, "PWM Rate":dbl}}
  T16 = typedef "WPI_MotorControlType.ctl" = enum16{"PWM", "CAN", "DIO PWM"}
  T17 = typedef "FPGA_DIOPWMChannel.ctl" = enum8{"PWM 0", "PWM 1", "PWM 2", "PWM 3", "PWM 4", "PWM 5", "PWM 6", "PWM 7", "PWM 8", "PWM 9", "PWM MXP 0", "PWM MXP 1", "PWM MXP 2", "PWM MXP 3", "PWM MXP 4", "PWM MXP 5", "PWM MXP 6", "PWM MXP 7", "PWM MXP 8", "PWM MXP 9", "Invalid"}
  T18 = typedef "WPI_PWMDeadband.ctl" = cluster{"Name":string, "maxPositivePwm":i32, "minPositivePwm":i32, "centerPwm":i32, "maxNegativePwm":i32, "minNegativePwm":i32, "angularRange":u16}
  T19 = typedef "FPGA_DIOChannel.ctl" = enum8{"DIO 0", "DIO 1", "DIO 2", "DIO 3", "DIO 4", "DIO 5", "DIO 6", "DIO 7", "DIO 8", "DIO 9", "DIO MXP 0", "DIO MXP 1", "DIO MXP 2", "DIO MXP 3", "DIO MXP 4", "DIO MXP 5", "DIO MXP 6", "DIO MXP 7", "DIO MXP 8", "DIO MXP 9", "DIO MXP 10", "DIO MXP 11", "DIO MXP 12", "DIO MXP 13", "DIO MXP 14", "DIO MXP 15", "SPI Port CS1", "SPI Port CS2", "SPI Port CS3", "SPI Port MISO", "SPI Port MOSI", "Invalid"}
  T20 = typedef "WPI_JoystickDevRef.ctl" = cluster{"Device":T21}
  T21 = typedef "WPI_JoystickDeviceEnum.ctl" = enum16{"USB 0", "USB 1", "USB 2", "USB 3", "USB 4", "USB 5"}
  T22 = enum16{"Do Nothing", "S - Scale Only", "O - Scale Only", "Middle Switch Two", "Middle Switch One", "Quarter Switch Only", "Outer Scale", "Cross"}
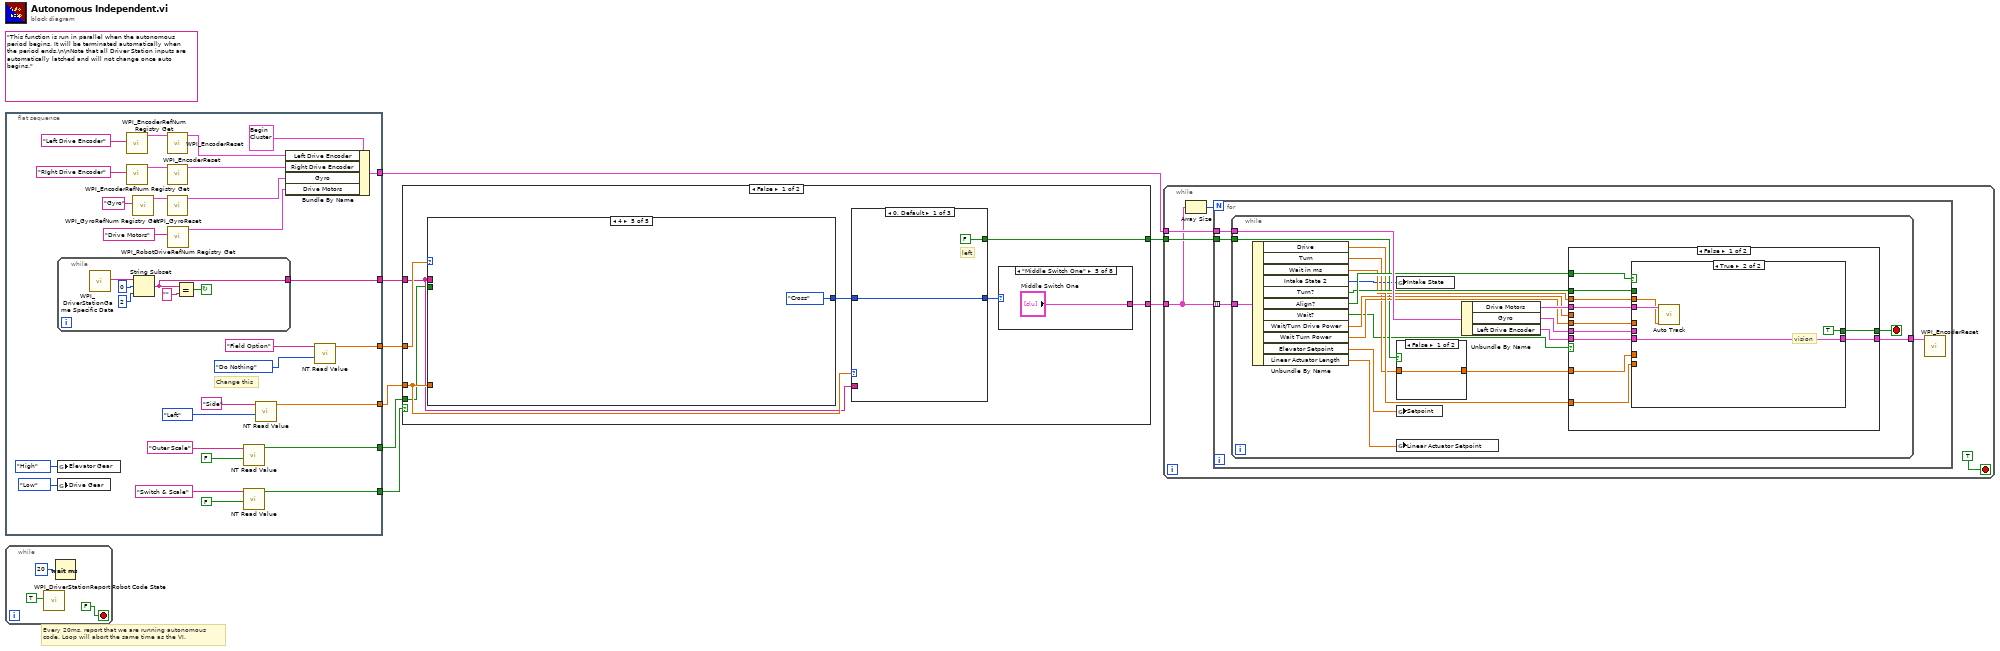
[diagram p0: block diagram]
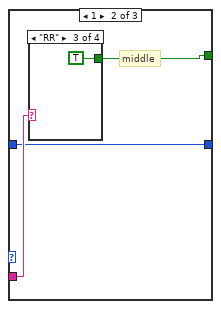
[diagram p2: hidden frame]
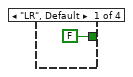
[diagram p3: hidden frame]
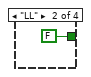
[diagram p4: hidden frame]
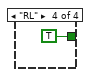
[diagram p5: hidden frame]
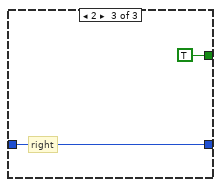
[diagram p6: hidden frame]
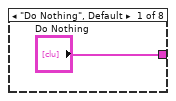
[diagram p7: hidden frame]
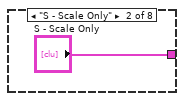
[diagram p8: hidden frame]
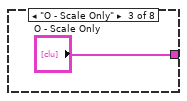
[diagram p9: hidden frame]
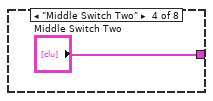
[diagram p10: hidden frame]
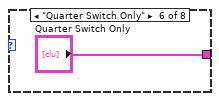
[diagram p11: hidden frame]
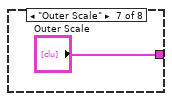
[diagram p12: hidden frame]
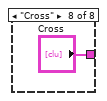
[diagram p13: hidden frame]
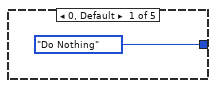
[diagram p14: hidden frame]
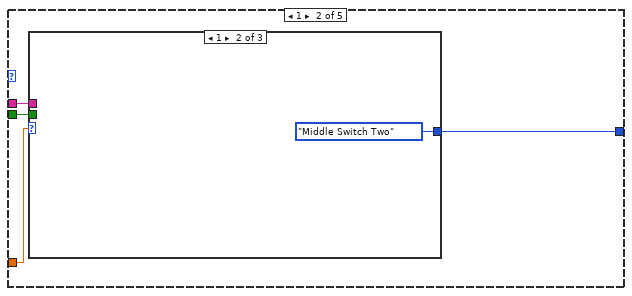
[diagram p15: hidden frame]
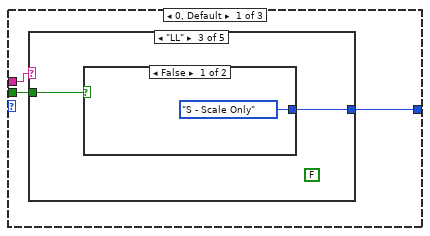
[diagram p16: hidden frame]
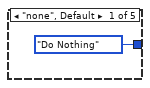
[diagram p17: hidden frame]
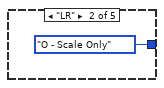
[diagram p18: hidden frame]
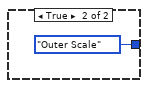
[diagram p19: hidden frame]
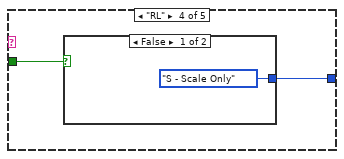
[diagram p20: hidden frame]
diagram:
  (unwired) "This function is run in parallel when the autonomous period begins. It will be terminated automatically when the period ends.\n\nNote that all Driver Station inputs are automatically latched and will not change once auto begins."
  # "Every 20ms, report that we are running autonomous\ncode. Loop will abort the same time as the VI."
  n1 = flat-sequence {
    tunnel: [w19] -> w8
    tunnel: [w23] -> w7
    tunnel: [w15] -> w5
    tunnel: [w16] -> w6
    tunnel: [w12] -> w3
    tunnel: [w11] -> w2
    frame #0 {
      # "Change this"
      n2 = while {
        tunnel: [w38] -> w15
        stop <- w39 continue-if-true
        n3 = call <vilib>:"WPI_DriverStationGame Specific Data.vi"() -> ("Game Specific Data"=w41:string)  [unwired: 11 in]
        n4 = String Subset(string=w41, offset (0)=0, length (rest)=2 ("length (rest)")) -> (substring=w38:string)
        n5 = Equal?(x=w38, y="") -> (x = y?=w39:bool)
      }
      n6 = global write "Global Variables.vi" "Elevator Gear"(enum16{"Low", "High"}."High" ("Drive Gear")) -> ()
      n7 = global write "Global Variables.vi" "Drive Gear"(enum16{"Low", "High"}."Low" ("Drive Gear")) -> ()
      n8 = call <vilib>:"WPI_EncoderRefNum Registry Get.vi"("refnum name"="Left Drive Encoder") -> ("EncoderDevRef"=w35:T4)  [unwired: 9 in, 1 out]
      n9 = call <vilib>:"WPI_EncoderRefNum Registry Get.vi"("refnum name"="RIght Drive Encoder") -> ("EncoderDevRef"=w32:T4)  [unwired: 9 in, 1 out]
      n10 = call <vilib>:"WPI_GyroRefNum Registry Get.vi"("refnum name"="Gyro") -> ("GyroDevRef"=w31:T12)  [unwired: 9 in, 1 out]
      n11 = call <vilib>:"WPI_EncoderReset.vi"("EncoderDevRef"=w35) -> ("EncoderDevRef"=w29:T4)  [unwired: 9 in, 1 out]
      n12 = call <vilib>:"WPI_EncoderReset.vi"("EncoderDevRef"=w32) -> ("EncoderDevRef"=w28:T4)  [unwired: 9 in, 1 out]
      n13 = call <vilib>:"WPI_GyroReset.vi"("GyroDevRef"=w31) -> ("GyroDevRef"=w27:T12)  [unwired: 9 in, 1 out]
      n14 = call <vilib>:"WPI_RobotDriveRefNum Registry Get.vi"("refnum name"="Drive Motors") -> ("RobotDriveDevRef"=w26:T14)  [unwired: 9 in, 1 out]
      n15 = call-poly <vilib>:"NT Read Value.vi"("Default Value"=FALSE, "Name"="Outer Scale") -> ("Boolean"=w12:bool)  [unwired: 8 in, 1 out]
      n16 = call-poly <vilib>:"NT Read Value.vi"("Default Value"=FALSE, "Name"="Switch & Scale") -> ("Boolean"=w11:bool)  [unwired: 8 in, 1 out]
      n17 = call-poly <vilib>:"NT Read Value.vi"("Default Value"=enum16{"Left", "Middle", "Right"}."Left", "Name"="Side") -> ("Numeric"=w16:dbl)  [unwired: 8 in, 1 out]
      n18 = Bundle By Name(cluster=T3 {"Left Drive Encoder"={"DevStatus"={"status"=FALSE, "code"=0, "source"=""}, "EncoderIndex"=enum."Invalid", "CounterIndex"=enum."Ctr 1", "DistancePerCount"=2.0, "Decoding Type"=enum."4x"}, "Right Drive Encoder"={"DevStatus"={"status"=FALSE, "code"=0, "source"=""}, "EncoderIndex"=enum."Invalid", "CounterIndex"=enum."Ctr 1", "DistancePerCount"=2.0, "Decoding Type"=enum."4x"}, "Elevator Encoder"={"DevStatus"={"status"=FALSE, "code"=0, "source"=""}, "EncoderIndex"=enum."Invalid", "CounterIndex"=enum."Ctr 1", "DistancePerCount"=2.0, "Decoding Type"=enum."4x"}, "Drive Shifter"={"DevStatus"={"status"=FALSE, "code"=0, "source"=""}, "Pneumatics Control Module"=0, "Forward Solenoid Channel"=enum."Invalid", "Reverse Solenoid Channel"=enum."Invalid"}, "Elevator Shifter"={"DevStatus"={"status"=FALSE, "code"=0, "source"=""}, "Pneumatics Control Module"=0, "Forward Solenoid Channel"=enum."Invalid", "Reverse Solenoid Channel"=enum."Invalid"}, "Elevator Brake"={"DevStatus"={"status"=FALSE, "code"=0, "source"=""}, "Pneumatics Control Module"=0, "Forward Solenoid Channel"=enum."Invalid", "Reverse Solenoid Channel"=enum."Invalid"}, "Intake Clamp"={"DevStatus"={"status"=FALSE, "code"=0, "source"=""}, "Pneumatics Control Module"=0, "Forward Solenoid Channel"=enum."Invalid", "Reverse Solenoid Channel"=enum."Invalid"}, "Intake Hinge"={"DevStatus"={"status"=FALSE, "code"=0, "source"=""}, "Pneumatics Control Module"=0, "Forward Solenoid Channel"=enum."Invalid", "Reverse Solenoid Channel"=enum."Invalid"}, "Pot Left"={"DevStatus"={"status"=FALSE, "code"=0, "source"=""}, "Analog Channel"=enum."Invalid", "Invert Output"=FALSE}, "Pot Right"={"DevStatus"={"status"=FALSE, "code"=0, "source"=""}, "Analog Channel"=enum."Invalid", "Invert Output"=FALSE}, "Gyro"={"DevStatus"={"status"=FALSE, "code"=0, "source"=""}, "Analog Channel"=enum."AI 1", "Gain (VoltsPerDegree/Second)"=0.0, "Gyro Type"=enum."Analog", "Handle"=0, "SPI Bus"=enum."Invalid", "Device Found"=FALSE, "Sample Rate"=1.0, "Calibrate On Open"=FALSE, "Offset"=0.0}, "Drive Motors"={"DevStatus"={"status"=FALSE, "code"=0, "source"=""}, "Motors[]"=[], "Square Inputs"=FALSE, "Max Output"=1.0}, "Elevator Master"={"DeviceStatus"={"status"=FALSE, "code"=0, "source"=""}, "Type"=enum."PWM", "PWM"={"PWM Channel"=enum."Invalid", "DeadBand"={"Name"="", "maxPositivePwm"=0, "minPositivePwm"=0, "centerPwm"=0, "maxNegativePwm"=0, "minNegativePwm"=0, "angularRange"=0}}, "CAN"={"Device Number"=0, "SetOutput VI Ref"=variant(refnum<vi> refnum), "GetOutput VI Ref"=variant(refnum<vi> refnum), "Enable VI Ref"=variant(refnum<vi> refnum), "Disable VI Ref"=variant(refnum<vi> refnum), "Data"=variant}, "Invert"=FALSE, "DIO PWM"={"PWM \"Enable\" Channel"=enum."Invalid", "DIOChannel"=enum."Invalid", "PWM Rate"=0.0}}, "Intake Left"={"DeviceStatus"={"status"=FALSE, "code"=0, "source"=""}, "Type"=enum."PWM", "PWM"={"PWM Channel"=enum."Invalid", "DeadBand"={"Name"="", "maxPositivePwm"=0, "minPositivePwm"=0, "centerPwm"=0, "maxNegativePwm"=0, "minNegativePwm"=0, "angularRange"=0}}, "CAN"={"Device Number"=0, "SetOutput VI Ref"=variant(refnum<vi> refnum), "GetOutput VI Ref"=variant(refnum<vi> refnum), "Enable VI Ref"=variant(refnum<vi> refnum), "Disable VI Ref"=variant(refnum<vi> refnum), "Data"=variant}, "Invert"=FALSE, "DIO PWM"={"PWM \"Enable\" Channel"=enum."Invalid", "DIOChannel"=enum."Invalid", "PWM Rate"=0.0}}, "Intake Right"={"DeviceStatus"={"status"=FALSE, "code"=0, "source"=""}, "Type"=enum."PWM", "PWM"={"PWM Channel"=enum."Invalid", "DeadBand"={"Name"="", "maxPositivePwm"=0, "minPositivePwm"=0, "centerPwm"=0, "maxNegativePwm"=0, "minNegativePwm"=0, "angularRange"=0}}, "CAN"={"Device Number"=0, "SetOutput VI Ref"=variant(refnum<vi> refnum), "GetOutput VI Ref"=variant(refnum<vi> refnum), "Enable VI Ref"=variant(refnum<vi> refnum), "Disable VI Ref"=variant(refnum<vi> refnum), "Data"=variant}, "Invert"=FALSE, "DIO PWM"={"PWM \"Enable\" Channel"=enum."Invalid", "DIOChannel"=enum."Invalid", "PWM Rate"=0.0}}, "Linear Actuator Left"={"DeviceStatus"={"status"=FALSE, "code"=0, "source"=""}, "Type"=enum."PWM", "PWM"={"PWM Channel"=enum."Invalid", "DeadBand"={"Name"="", "maxPositivePwm"=0, "minPositivePwm"=0, "centerPwm"=0, "maxNegativePwm"=0, "minNegativePwm"=0, "angularRange"=0}}, "CAN"={"Device Number"=0, "SetOutput VI Ref"=variant(refnum<vi> refnum), "GetOutput VI Ref"=variant(refnum<vi> refnum), "Enable VI Ref"=variant(refnum<vi> refnum), "Disable VI Ref"=variant(refnum<vi> refnum), "Data"=variant}, "Invert"=FALSE, "DIO PWM"={"PWM \"Enable\" Channel"=enum."Invalid", "DIOChannel"=enum."Invalid", "PWM Rate"=0.0}}, "Linear Actuator Right"={"DeviceStatus"={"status"=FALSE, "code"=0, "source"=""}, "Type"=enum."PWM", "PWM"={"PWM Channel"=enum."Invalid", "DeadBand"={"Name"="", "maxPositivePwm"=0, "minPositivePwm"=0, "centerPwm"=0, "maxNegativePwm"=0, "minNegativePwm"=0, "angularRange"=0}}, "CAN"={"Device Number"=0, "SetOutput VI Ref"=variant(refnum<vi> refnum), "GetOutput VI Ref"=variant(refnum<vi> refnum), "Enable VI Ref"=variant(refnum<vi> refnum), "Disable VI Ref"=variant(refnum<vi> refnum), "Data"=variant}, "Invert"=FALSE, "DIO PWM"={"PWM \"Enable\" Channel"=enum."Invalid", "DIOChannel"=enum."Invalid", "PWM Rate"=0.0}}, "X Joystick"={"Device"=enum."USB 1"}, "Y Joystick"={"Device"=enum."USB 1"}, "Controller"={"Device"=enum."USB 1"}, "775 Drive Motors"={"DevStatus"={"status"=FALSE, "code"=0, "source"=""}, "Motors[]"=[], "Square Inputs"=FALSE, "Max Output"=1.0}, "Intake Angle Encoder"={"DevStatus"={"status"=FALSE, "code"=0, "source"=""}, "EncoderIndex"=enum."Invalid", "CounterIndex"=enum."Ctr 1", "DistancePerCount"=2.0, "Decoding Type"=enum."4x"}, "Intake Angle"={"DeviceStatus"={"status"=FALSE, "code"=0, "source"=""}, "Type"=enum."PWM", "PWM"={"PWM Channel"=enum."Invalid", "DeadBand"={"Name"="", "maxPositivePwm"=0, "minPositivePwm"=0, "centerPwm"=0, "maxNegativePwm"=0, "minNegativePwm"=0, "angularRange"=0}}, "CAN"={"Device Number"=0, "SetOutput VI Ref"=variant(refnum<vi> refnum), "GetOutput VI Ref"=variant(refnum<vi> refnum), "Enable VI Ref"=variant(refnum<vi> refnum), "Disable VI Ref"=variant(refnum<vi> refnum), "Data"=variant}, "Invert"=FALSE, "DIO PWM"={"PWM \"Enable\" Channel"=enum."Invalid", "DIOChannel"=enum."Invalid", "PWM Rate"=0.0}}} ("Begin Cluster"), "Left Drive Encoder"=w29, "Right Drive Encoder"=w28, "Gyro"=w27, "Drive Motors"=w26) -> (w23:T3)
      n19 = call-poly <vilib>:"NT Read Value.vi"("Default Value"=T2."Do Nothing", "Name"="Field Option") -> ("Numeric"=w19:dbl)  [unwired: 8 in, 1 out]
    }
  }
  n20 = while {
    stop <- FALSE stop-if-true
    n21 = call <vilib>:"WPI_DriverStationReport Robot Code State.vi"("Autonomous"=TRUE) -> ()  [unwired: 10 in, 1 out]
    n22 = Wait (ms)(milliseconds to wait=u32 20) -> ()  [unwired: 1 out]
  }
  n23 = case shown="False" w2 {
    tunnel: w8 -> [w53 _]
    tunnel: w6 -> [w52 w151]
    tunnel: w5 -> [w51 w149]
    tunnel: [w50 w150] -> w4
    tunnel: [w47 w147] -> w1
    tunnel: w3 -> [w46 _]
    frame False {
      n24 = case shown="4" w53 {
        tunnel: w51 -> [_ w77 w109 w142 _]
        tunnel: w52 -> [_ w76 w110 w141 _]
        tunnel: [T22."Do Nothing" w75 w108 w140 T22."Cross"] -> w48
        tunnel: w46 -> [_ w74 w107 _ _]
        frame 0, Default {
        }
        frame 1 {
          n25 = case shown="1" w76 {
            tunnel: w77 -> [w80 _ w95]
            tunnel: [w79 T22."Middle Switch Two" w94] -> w75
            tunnel: w74 -> [w78 _ w93]
            frame 0, Default {
              n26 = case shown="\"LL\"" w80 {
                tunnel: [T22."Do Nothing" T22."O - Scale Only" w83 w87 T22."O - Scale Only"] -> w79
                tunnel: w78 -> [_ _ w84 w88 _]
                frame "none", Default {
                }
                frame "LR" {
                }
                frame "LL" {
                  (unwired) FALSE
                  n27 = case shown="False" w84 {
                    tunnel: [T22."S - Scale Only" T22."Outer Scale"] -> w83
                    frame False {
                    }
                    frame True {
                    }
                  }
                }
                frame "RL" {
                  n28 = case shown="False" w88 {
                    tunnel: [T22."S - Scale Only" T22."Outer Scale"] -> w87
                    frame False {
                    }
                    frame True {
                    }
                  }
                }
                frame "RR" {
                  (unwired) FALSE
                }
              }
            }
            frame 1 {
            }
            frame 2 {
              n29 = case shown="\"LL\"" w95 {
                tunnel: [T22."Do Nothing" w97 T22."O - Scale Only" T22."O - Scale Only" w104] -> w94
                tunnel: w93 -> [_ w98 _ _ w103]
                frame "none", Default {
                }
                frame "LR" {
                  n30 = case shown="False" w98 {
                    tunnel: [T22."S - Scale Only" T22."Outer Scale"] -> w97
                    frame False {
                    }
                    frame True {
                    }
                  }
                }
                frame "LL" {
                }
                frame "RL" {
                }
                frame "RR" {
                  n31 = case shown="True" w103 {
                    tunnel: [T22."S - Scale Only" T22."Outer Scale"] -> w104
                    frame False {
                    }
                    frame True {
                    }
                  }
                }
              }
            }
          }
        }
        frame 2 {
          n32 = case shown="1" w110 {
            tunnel: w109 -> [w113 _ w127]
            tunnel: [w112 T22."Middle Switch One" w128] -> w108
            tunnel: w107 -> [w111 _ w126]
            frame 0, Default {
              n33 = case shown="\"none\", Default" w113 {
                tunnel: [T22."Do Nothing" T22."Quarter Switch Only" w117 w120 T22."Cross"] -> w112
                tunnel: w111 -> [_ _ w116 w121 _]
                frame "none", Default {
                }
                frame "LR" {
                }
                frame "LL" {
                  n34 = case shown="False" w116 {
                    tunnel: [T22."S - Scale Only" T22."Outer Scale"] -> w117
                    frame False {
                    }
                    frame True {
                    }
                  }
                }
                frame "RL" {
                  n35 = case shown="False" w121 {
                    tunnel: [T22."S - Scale Only" T22."Outer Scale"] -> w120
                    frame False {
                    }
                    frame True {
                    }
                  }
                }
                frame "RR" {
                }
              }
            }
            frame 1 {
            }
            frame 2 {
              n36 = case shown="\"RR\"" w127 {
                tunnel: [T22."Do Nothing" w130 T22."Cross" T22."Quarter Switch Only" w136] -> w128
                tunnel: w126 -> [_ w131 _ _ w137]
                frame "none", Default {
                }
                frame "LR" {
                  n37 = case shown="False" w131 {
                    tunnel: [T22."S - Scale Only" T22."Outer Scale"] -> w130
                    frame False {
                    }
                    frame True {
                    }
                  }
                }
                frame "LL" {
                }
                frame "RL" {
                }
                frame "RR" {
                  n38 = case shown="False" w137 {
                    tunnel: [T22."S - Scale Only" T22."Outer Scale"] -> w136
                    frame False {
                    }
                    frame True {
                    }
                  }
                }
              }
            }
          }
        }
        frame 3 {
          n39 = case shown="1" w141 {
            tunnel: w142 -> [_ _ _]
            tunnel: [T22."Quarter Switch Only" T22."Middle Switch Two" T22."Quarter Switch Only"] -> w140
            frame 0, Default {
            }
            frame 1 {
            }
            frame 2 {
            }
          }
        }
        frame 4 {
        }
      }
      n40 = case shown="0, Default" w52 {
        tunnel: w51 -> [_ w58 _]
        tunnel: [FALSE w57 TRUE] -> w50
        tunnel: w48 -> [w54 w56 w63]
        tunnel: [w54 w56 w63] -> w49
        frame 0, Default {
          # "left"
        }
        frame 1 {
          # "middle"
          n41 = case shown="\"RR\"" w58 {
            tunnel: [FALSE FALSE TRUE TRUE] -> w57
            frame "LR", Default {
            }
            frame "LL" {
            }
            frame "RR" {
            }
            frame "RL" {
            }
          }
        }
        frame 2 {
          # "right"
        }
      }
      n42 = case shown="\"Middle Switch One\"" w49 {
        tunnel: ["Do Nothing" "S - Scale Only" "O - Scale Only" "Middle Switch Two" "Middle Switch One" "Quarter Switch Only" "Outer Scale" "Cross"] -> w47
        frame "Do Nothing", Default {
        }
        frame "S - Scale Only" {
        }
        frame "O - Scale Only" {
        }
        frame "Middle Switch Two" {
        }
        frame "Middle Switch One" {
        }
        frame "Quarter Switch Only" {
        }
        frame "Outer Scale" {
        }
        frame "Cross" {
        }
      }
    }
    frame True {
      n43 = case shown="2" w151 {
        tunnel: [FALSE TRUE TRUE] -> w150
        tunnel: w149 -> [w156 _ w167]
        tunnel: [w157 enum16{"OO", "OS", "SO", "SS"}."SS" w166] -> w148
        frame 0, Default {
          n44 = case shown="\"RR\", Default" w156 {
            tunnel: [enum16{"OO", "OS", "SO", "SS"}."OO" enum16{"OO", "OS", "SO", "SS"}."OS" enum16{"OO", "OS", "SO", "SS"}."SO" enum16{"OO", "OS", "SO", "SS"}."SS"] -> w157
            frame "RR", Default {
            }
            frame "RL" {
            }
            frame "LR" {
            }
            frame "LL" {
            }
          }
        }
        frame 1 {
        }
        frame 2 {
          n45 = case shown="\"LL\"" w167 {
            tunnel: [enum16{"OO", "OS", "SO", "SS"}."SS" enum16{"OO", "OS", "SO", "SS"}."SO" enum16{"OO", "OS", "SO", "SS"}."OS" enum16{"OO", "OS", "SO", "SS"}."OO"] -> w166
            frame "RR", Default {
            }
            frame "RL" {
            }
            frame "LR" {
            }
            frame "LL" {
            }
          }
        }
      }
      n46 = case shown="\"OO\"" w148 {
        tunnel: ["OS - Switch & Scale" "SO - Switch & Scale" "SS - Switch & Scale" "OO - Switch & Scale"] -> w147
        frame "OS", Default {
        }
        frame "SO" {
        }
        frame "SS" {
        }
        frame "OO" {
        }
      }
    }
  }
  n47 = while {
    tunnel: w7 -> [w174]
    tunnel: w4 -> [w173]
    tunnel: w1 -> [w172]
    stop <- TRUE stop-if-true
    n48 = Array Size(array=w172) -> (size(s)=w175:i32)
    n49 = for {
      N: w175 -> [_]
      tunnel: w174 -> [w180]
      tunnel: w173 -> [w178]
      tunnel: w172 -> [w177] mode=indexing
      n50 = while {
        tunnel: w180 -> [w200]
        tunnel: [w199] -> w179
        tunnel: w178 -> [w186]
        tunnel: w177 -> [w185]
        stop <- w192 stop-if-true
        n51 = Unbundle By Name(w185) -> ("Drive"=w193:dbl, "Turn"=w188:dbl, "Wait in ms"=w191:dbl, "Intake State 2"=w181:enum16{"Off", "Intake", "Spit Low", "Spit High"}, "Turn?"=w197:bool, "Align?"=w198:bool, "Wait?"=w184:bool, "Wait/Turn Drive Power"=w190:dbl, "Wait Turn Power"=w189:dbl, "Elevator Setpoint"=w183:dbl, "Linear Actuator Length"=w182:dbl)
        n52 = global write "Global Variables.vi" "Intake State"(w181) -> ()
        n53 = case shown="False" w186 {
          tunnel: w188 -> [w201 w202]
          tunnel: [w201 w203] -> w187
          frame False {
          }
          frame True {
            n54 = Negate(x=w202) -> (-x=w203:dbl)
          }
        }
        n55 = global write "Global Variables.vi" "Setpoint"(w183) -> ()
        n56 = global write "Global Variables.vi" "Linear Actuator Setpoint"(w182) -> ()
        n57 = Unbundle By Name(w200) -> ("Drive Motors"=w196:T14, "Gyro"=w195:T12, "Left Drive Encoder"=w194:T4)
        n58 = case shown="False" w184 {
          tunnel: w196 -> [w214 w244]
          tunnel: w195 -> [w213 _]
          tunnel: w194 -> [w212 w245]
          tunnel: [w211 w245] -> w199
          tunnel: w198 -> [w205 _]
          tunnel: w197 -> [w210 _]
          tunnel: w187 -> [w209 _]
          tunnel: w193 -> [w208 _]
          tunnel: [w207 TRUE ("In Range?")] -> w192
          tunnel: w191 -> [w204 w243]
          tunnel: w190 -> [_ w242]
          tunnel: w189 -> [w206 w241]
          frame False {
            n59 = case shown="True" w205 {
              tunnel: w214 -> [w223 w238]
              tunnel: w213 -> [w222 _]
              tunnel: w212 -> [w221 w239]
              tunnel: [w220 w239] -> w211
              tunnel: w210 -> [w215 _]
              tunnel: w209 -> [w219 _]
              tunnel: w208 -> [w218 _]
              tunnel: [w216 TRUE] -> w207
              tunnel: w206 -> [w217 _]
              tunnel: w204 -> [_ w237]
              frame False {
                n60 = case shown="True" w215 {
                  tunnel: w223 -> [w230 w236]
                  tunnel: w222 -> [w229 w235]
                  tunnel: w221 -> [w228 w233]
                  tunnel: [w227 w233] -> w220
                  tunnel: w219 -> [w226 w234]
                  tunnel: w218 -> [w224 _]
                  tunnel: w217 -> [_ w231]
                  tunnel: [w225 w232] -> w216
                  frame False {
                    # "regular drive"
                    n61 = call "Auto Drive.vi"("Drive Dev Ref in"=w230, "Gyro Dev Ref in"=w229, "Encoder Dev Ref in"=w228, "X setpoint"=w226, "Y setpoint"=w224) -> ("Encoder Dev Ref out"=w227:T4, "In Range?"=w225:bool)  [unwired: 6 in, 3 out]
                  }
                  frame True {
                    # "regular turn"
                    n62 = call "Auto Turn.vi"("X setpoint"=w234, "Y axis value"=w231, "Gyro Dev Ref in"=w235, "Drive Dev Ref in"=w236) -> ("In Range?"=w232:bool)  [unwired: 4 in, 3 out]
                  }
                }
              }
              frame True {
                # "vision"
                n63 = call "Auto Track.vi"("wait"=w237, "Drive Dev Ref in"=w238) -> ()  [unwired: 9 in, 1 out]
              }
            }
          }
          frame True {
            n64 = Wait (ms)(milliseconds to wait=w243) -> ()  [unwired: 1 out]
            n65 = call-poly <vilib>:"WPI_RobotDriveArcadeDrive.vi"("Y axis value"=w242, "X axis value"=w241, "RobotDriveDevRef"=w244) -> ()  [unwired: 6 in, 3 out]
          }
        }
      }
      n66 = call <vilib>:"WPI_EncoderReset.vi"("EncoderDevRef"=w179) -> ()  [unwired: 9 in, 2 out]
    }
  }
